vi "Translator.vi"(0 "Input":variant, 11 "error in (no error)":errorcluster) -> (4 "Output":variant, 15 "error out":errorcluster)   [LabVIEW 2014]
doc: "An example of how to create the Translator to convert the LabVIEW VIs to Arduino C code."
panel:
  out "Outputs":string[](array[string])
  out "Inputs":string[](array[string])
  out "Output Datatypes":string[](array[string])
  out "Input Datatypes":string[](array[string])
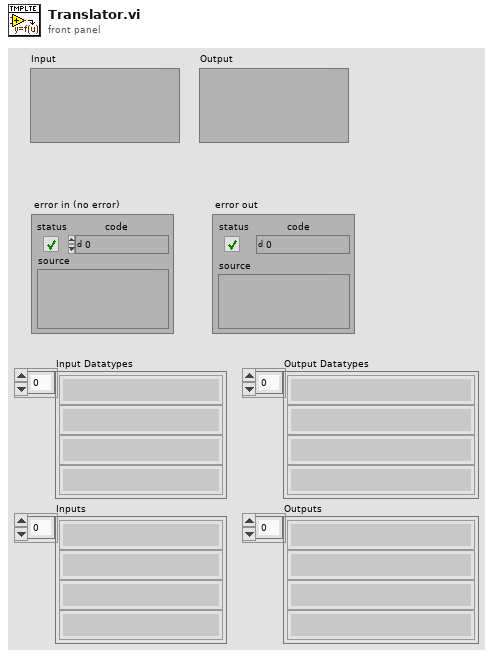
[diagram p1: front panel]
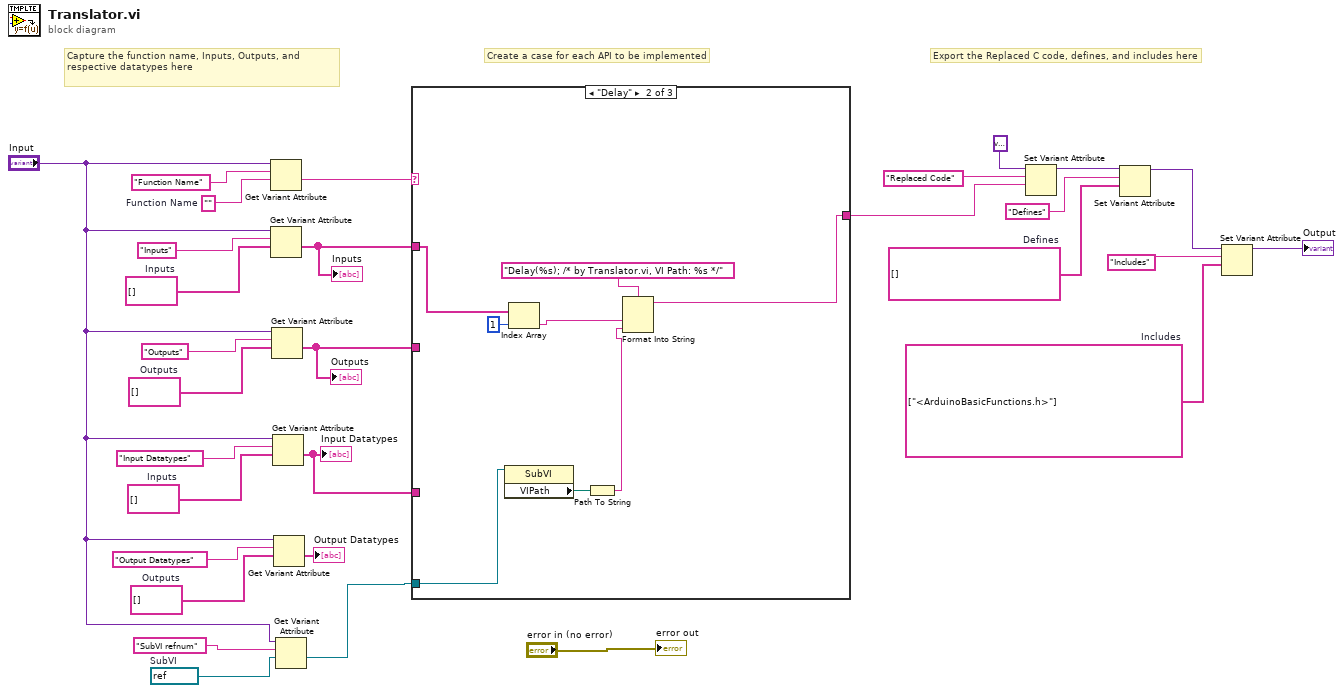
[diagram p0: block diagram]
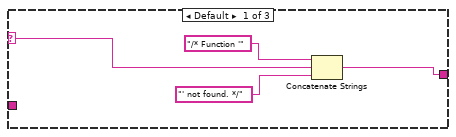
[diagram p2: hidden frame]
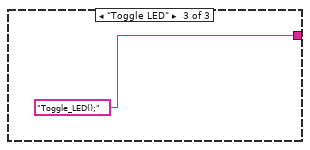
[diagram p3: hidden frame]
diagram:
  w2 = refnum<vi> refnum  # SubVI
  w6 = string[] []  # Defines
  w15 = string[] []  # Outputs
  w16 = string[] []  # Inputs
  w21 = string[] ["<ArduinoBasicFunctions.h>"]  # Includes
  w26 = string[] []  # Outputs
  w27 = string[] []  # Inputs
  w28 = ""  # Function Name
  # "Capture the function name, Inputs, Outputs, and respective datatypes here"
  # "Export the Replaced C code, defines, and includes here"
  # "Create a case for each API to be implemented"
  n1 = Get Variant Attribute(Variant="Input", name="Function Name", default value (empty Variant)=w28) -> (value=w23:string)  [unwired: 1 in, 3 out]
  n2 = Get Variant Attribute(Variant="Input", name="Inputs", default value (empty Variant)=w27) -> (value=w11:string[])  [unwired: 1 in, 3 out]
  "Inputs" <- w11
  n3 = Get Variant Attribute(Variant="Input", name="Outputs", default value (empty Variant)=w26) -> (value=w12:string[])  [unwired: 1 in, 3 out]
  "Outputs" <- w12
  n4 = Get Variant Attribute(Variant="Input", name="Input Datatypes", default value (empty Variant)=w16) -> (value=w5:string[])  [unwired: 1 in, 3 out]
  "Input Datatypes" <- w5
  n5 = Get Variant Attribute(Variant="Input", name="Output Datatypes", default value (empty Variant)=w15) -> (value=→"Output Datatypes":string[])  [unwired: 1 in, 3 out]
  n6 = Get Variant Attribute(Variant="Input", name="SubVI refnum", default value (empty Variant)=w2) -> (value=w1:refnum<vi>)  [unwired: 1 in, 3 out]
  n7 = case shown="\"Delay\"" w23 {
    selector: w23 -> [w33 _ _]
    tunnel: [w31 w38 "Toggle_LED();" ("format string")] -> w22
    tunnel: w11 -> [_ w41 _]
    tunnel: w12 -> [_ _ _]
    tunnel: w5 -> [_ _ _]
    tunnel: w1 -> [_ w37 _]
    frame Default {
      n8 = Concatenate Strings("/* Function '", w33, "' not found. */") -> (w31:string)
    }
    frame "Delay" {
      n9 = property class="SubVI"(reference=w37) -> ("VIPath"=w36:path)  [unwired: 1 in, 2 out]
      n10 = Index Array(array=w41, index=1) -> (element=w40:string)
      n11 = Path To String(path=w36) -> (string=w35:string)
      n12 = Format Into String(format string="Delay(%s); /* by Translator.vi, VI Path: %s */", w40, w35) -> (resulting string=w38:string)  [unwired: 2 in, 1 out]
    }
    frame "Toggle LED" {
    }
  }
  n13 = Set Variant Attribute(Variant=variant ("variant"), name="Replaced Code", value=w22) -> (Variant out=w9:variant)  [unwired: 1 in, 2 out]
  n14 = Set Variant Attribute(Variant=w9, name="Defines", value=w6) -> (Variant out=w8:variant)  [unwired: 1 in, 2 out]
  n15 = Set Variant Attribute(Variant=w8, name="Includes", value=w21) -> (Variant out=→"Output":variant)  [unwired: 1 in, 2 out]
  "error out" <- "error in (no error)"
